vi "Validate Condition.vi"(10 "Previous Condition":string, 11 "Condition in":string) -> (3 "Valid Condition out":string)   [LabVIEW 2020, in "Output Sequencer.lvlib" / "Settings UI.lvclass"]
uses:
  Settings UI.lvclass
  <vilib>/LAVA/muParser/mupExpr/mupExpr.lvclass
  Globals/Dialog Strings.vi
  Output Sequencer/Output Sequencer.lvclass
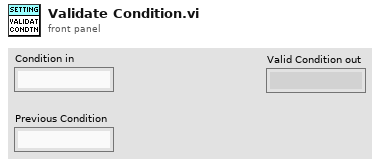
[diagram p1: front panel]
types:
  T1 = cluster{"error code":i32, "error message":string, "error pos":i32, "error token":string}
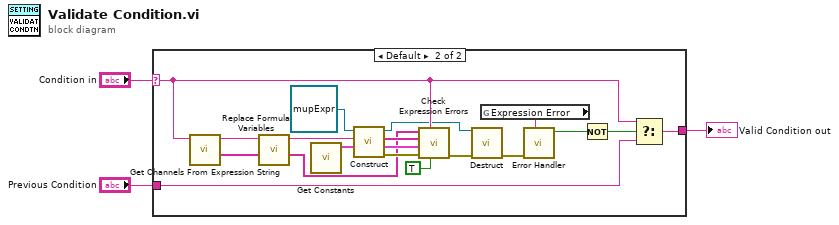
[diagram p0: block diagram]
diagram:
  n1 = case shown="Default" "Condition in" {
    selector: "Condition in" -> [w4 w21]
    tunnel: [w4 w23] -> w2
    tunnel: "Previous Condition" -> [_ w22]
    frame "" {
      # "Empty condition is always valid"
    }
    frame Default {
      n2 = call "Get Channels From Expression String.vi"("Expression String in"=w21) -> ("Channels (with quotes)"=w17:string[], "Expression String out"=w20:string)  [unwired: 7 in, 2 out]
      n3 = call "Replace Formula Variables.vi"("Variables to be replaced"=w17, "Formula in"=w20) -> ("Formula variables"=w9:string[], "Formula out"=w18:string)  [unwired: 7 in, 1 out]
      n4 = call "Get Constants.vi"() -> ("Constants"=w15:cluster{"name":string, "value":dbl}[])  [unwired: 11 in]
      n5 = call-dynamic "Construct.vi"("Constants"=w15, "Expression"=w18, "muExpr in"=refnum<class "mupExpr.lvclass"> refnum) -> ("error out"=w14:errorcluster, "error details"=w13:T1, "Variable Names"=w12:string[], "mupExpr out"=w16:refnum<class "mupExpr.lvclass">)  [unwired: 5 in]
      n6 = call "Check Expression Errors.vi"("For dialog?"=TRUE, "Expression String in"=w21, "error in (no error)"=w14, "Parser Error Details"=w13, "Found Variables"=w12, "Expected Variables"=w9) -> ("error out"=w10:errorcluster)  [unwired: 5 in]
      n7 = call-dynamic "Destruct.vi"("error in (no error)"=w10, "muExpr in"=w16) -> ("error out"=w8:errorcluster)  [unwired: 9 in]
      n8 = global read "Dialog Strings.vi" "Expression Error"() -> (w6:string)
      n9 = call "Error Handler.vi"("Dialog Title (\"\")"=w6, "error in (no error)"=w8) -> ("Error?"=w7:bool)  [unwired: 9 in]
      n10 = Not(x=w7) -> (.not. x?=w11:bool)
      n11 = Select(t=w21, s=w11, f=w22) -> (s? t:f=w23:string)
    }
  }
  "Valid Condition out" <- w2
